vi "ALTS-2015 LV2GBL Restart Notifier Ref.vi"(7 "Options":T1, 8 "Error In":errorcluster, 9 "Authenticated User Name":string="Authenticated User Name", 11 "Restart Notifier In":refnum<notifier>) -> (0 "Error Out":errorcluster, 1 "Authenticated User Name Out":string="Authenticated User Name", 3 "Restart Notifier Out":refnum<notifier>)   [LabVIEW 2013]
uses:
  Controls/ALTS-2015 LV2GBL Restart Options.ctl
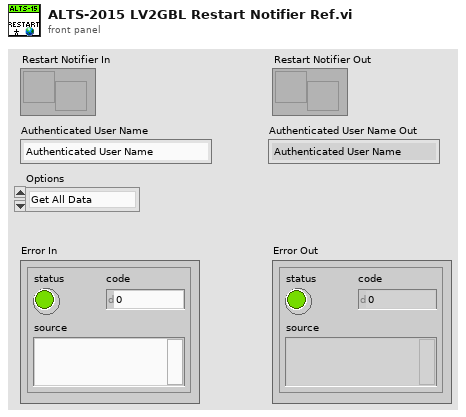
[diagram p1: front panel]
types:
  T1 = typedef "ALTS-2015 LV2GBL Restart Options.ctl" = enum16{"Get All Data", "Set Restart Notifier Ref", "Store Authentication Data"}
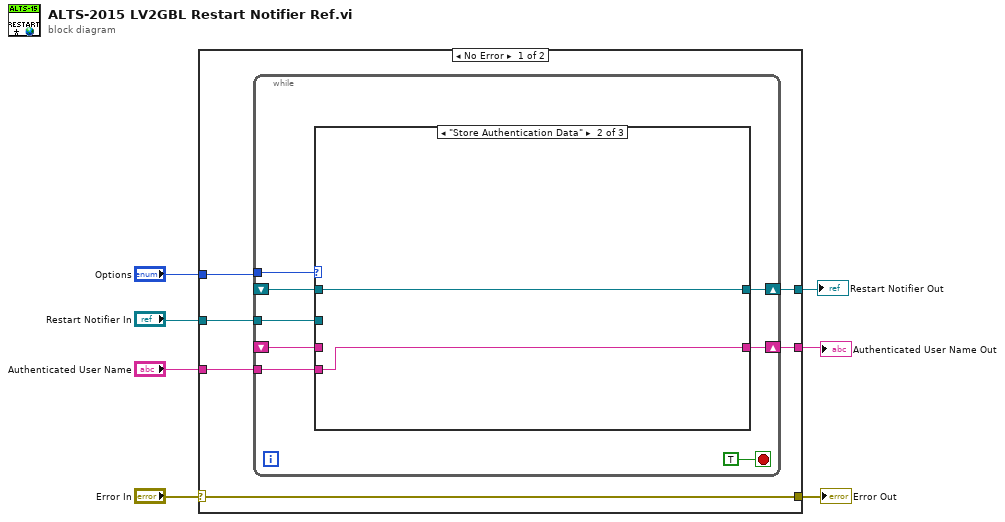
[diagram p0: block diagram]
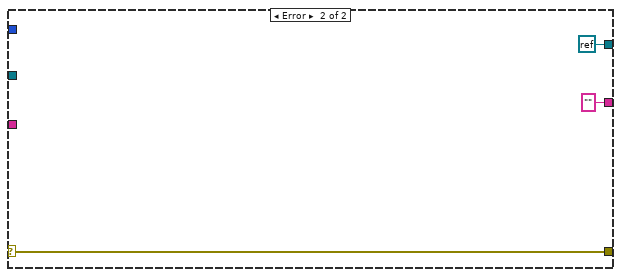
[diagram p4: hidden frame]
diagram:
  n1 = case shown="No Error" "Error In" {
    selector: "Error In" -> [w11 w29]
    tunnel: "Restart Notifier In" -> [w13 _]
    tunnel: [w12 refnum<k0> refnum] -> w4
    tunnel: [w11 w29] -> w6
    tunnel: "Options" -> [w10 _]
    tunnel: "Authenticated User Name" -> [w9 _]
    tunnel: [w8 "" ("Authenticated User Name")] -> w1
    frame No Error {
      n2 = while {
        tunnel: w10 -> [w20]
        tunnel: w13 -> [w18]
        shift-right: [w19] -> w12
        shift-left: _ -> [w17]
        tunnel: w9 -> [w15]
        shift-right: [w16] -> w8
        shift-left: _ -> [w14]
        stop <- TRUE stop-if-true
        n3 = case shown="\"Store Authentication Data\"" w20 {
          tunnel: [w23 w25 w27] -> w19
          tunnel: w18 -> [w23 _ _]
          tunnel: w17 -> [_ w25 w27]
          tunnel: [w22 w24 w26] -> w16
          tunnel: w15 -> [w22 w24 _]
          tunnel: w14 -> [_ _ w26]
          frame "Set Restart Notifier Ref" {
          }
          frame "Store Authentication Data" {
          }
          frame "Get All Data" {
          }
        }
      }
    }
    frame Error {
    }
  }
  "Error Out" <- w6
  "Restart Notifier Out" <- w4
  "Authenticated User Name Out" <- w1
